vi "Read Assigned Value.vi"(8 "error in (no error)":errorcluster, 11 "Assign abs_Value in":refnum<class "Assign abs_Value.lvclass">) -> (0 "error out":errorcluster, 2 "Abs_Value.lvclass":refnum<class "Abs_Value.lvclass">, 3 "Assign abs_Value out":refnum<class "Assign abs_Value.lvclass">)   [LabVIEW 2021, in "BT.lvlib" / "Assign abs_Value.lvclass"]
uses:
  Assign abs_Value.lvclass
  <vilib>/TSA/Abstract Data Classes/Abs_Types/Value/Abs_Value.lvclass
  Assign abs_Value.lvclass/Assign abs_Value.ctl
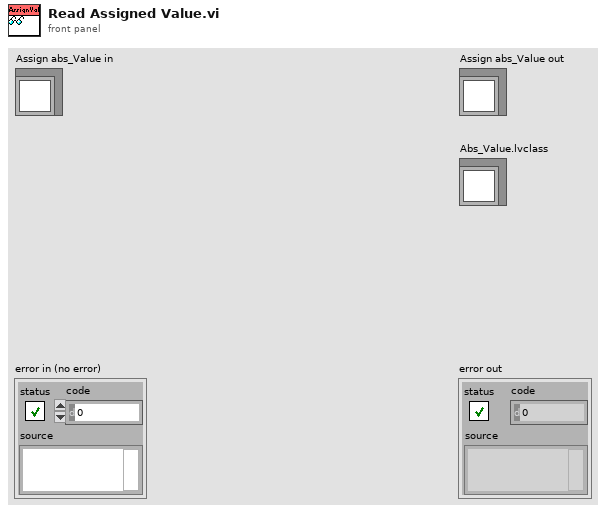
[diagram p1: front panel]
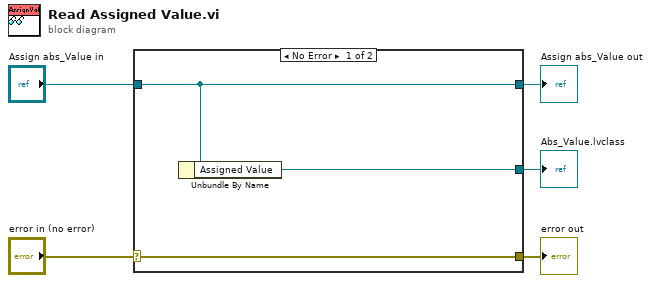
[diagram p0: block diagram]
diagram:
  n1 = case shown="No Error" "error in (no error)" {
    selector: "error in (no error)" -> [w8 w9]
    tunnel: [w8 w9] -> w4
    tunnel: [w7 w10] -> w2
    tunnel: "Assign abs_Value in" -> [w7 w10]
    tunnel: [w6 _] -> w1
    frame No Error {
      n2 = Unbundle By Name(w7) -> ("Assigned Value"=w6:refnum<class "Abs_Value.lvclass">)
    }
    frame Error {
    }
  }
  "error out" <- w4
  "Assign abs_Value out" <- w2
  "Abs_Value.lvclass" <- w1
